vi "Source A.vi"() -> ()   [LabVIEW 2016, in "beamline sections.lvlib"]
doc: "This vi allows the user to control the beamline elements on the high voltage deck. It uses the GRoup3 controllers to access all three high voltage decks. The preacc and injector image faraday cup are controlled by the low end compact rio"
uses:
  beamline sections.lvlib
  Users/wymanm/Desktop/Control computer - Copy/control/control vi/ion Source/Ion Source/ion source llb.lvlib
panel:
  in  "Tab Control":enum32{"Controls", "Readbacks"}(tab)
  out "Boolean":bool
  in  "Oven i":dbl
  in  "Y Steerer":dbl(knob) scale=-500.0..300.0
  in  "Pre-Acc":dbl(knob) scale=60.0..63.0
  in  "source 2 Einzel":dbl(knob) scale=4.0..10.0
  in  "X Steerer":dbl(knob) scale=300.0..-300.0
  in  "Source 1 Einzel":dbl(knob) scale=8.0..12.0
  in  "Extractor p":dbl(knob) scale=20.0..26.0
  in  "Immersion Lens":dbl(knob) scale=0.0..1.0
  out "Einzel 2":bool
  out "Cathode":bool
  out "Extractor":bool
  out "Oven":bool
  out "Immersion lens":bool
  out "Einzel 1":bool
  out "Steerer":bool
  out "Pre acc":bool=TRUE
  in  "Cathode vol":dbl(knob) scale=0.0..10.0
  out "Cathode  cluster":T1 {"Cathode" format="%#_3g"; "Cathode\nVoltage" format="%#.2g"; "Cathode \nCurrent" format="%#.2g"}
  out "Extractor  cluster":T2 {"Extractor" format="%#_3g"; "Extractor \nVoltage" format="%#.2g"; "Extractor\n Current" format="%#.2g"}
  out "Immersion Lens  cluster":T3 {"Immersion Lens" format="%#_3g"; "Immersion Lens\nCurrent" format="%#.2g"; "Immersion Lens\nVoltage" format="%#.2g"}
  in  "stop":bool
  out "Oven cluster":T4 {"Oven V" format="%#.2g"; "Oven power" format="%#.2g"; "Oven  I readback" format="%#.2g"; "Oven Current\n Set point" format="%#.2g"}
  out "Einzel 1  cluster":T5 {"Einzel 1\nVoltage" format="%#.2g"; "Einzel \nCurrent" format="%#.2g"}
  out "Source Steerer cluster":T6 {"X steerer" format="%#.2g"; "Y Steerer" format="%#.2g"}
  out "Einzel 2  cluster":T7 {"Einzel 2\nvoltage" format="%#.2g"; "Einzel 2 \nCurrent" format="%#.2g"}
  out "Preacc cluster":T8 {"Pre-acc Voltage" format="%#.2g"; "Pre-acc current" format="%#.2g"}
  out "Cryo pump":T9
  out "Ion gauge Cluster 1":T10
  out "cathode on?":bool
  out "sample change finished change":bool
  out "holder position":bool
  out "cathode on":bool
  out "chop voltage":dbl
  in  "reset oven":bool
  out "Ion Source Readbacks":dbl[][](array[numeric])
  out "Ion Source":dbl[][](array[numeric])
  out "Oven":dbl[](array[numeric])
  out "Einzel":dbl[](array[numeric])
  out "pre-acc set":dbl format="%#_3g"
  out "Pre-acc Voltage":dbl format="%#_3g"
  out "Pre-acc current":dbl format="%#_3g"
  out "inj cup out":bool
  out "Output Current":dbl format="%.4f"
  out "Output Power":dbl format="%.4f"
  out "Output Voltage":dbl format="%.4f"
  out "error out 2":errorcluster
  out "Read Set Current":dbl format="%.4f"
  out "Read Set Voltage":dbl format="%.4f"
  out "error out":errorcluster
  out "ID responce":string
  out "Address \"OK\"":string
  in  "Einzel 1  cluster 2":T5 {"Einzel 1\nVoltage" format="%#.2g"; "Einzel \nCurrent" format="%#.2g"}
  # "red is in the beamline\nblue is out of the beamline"
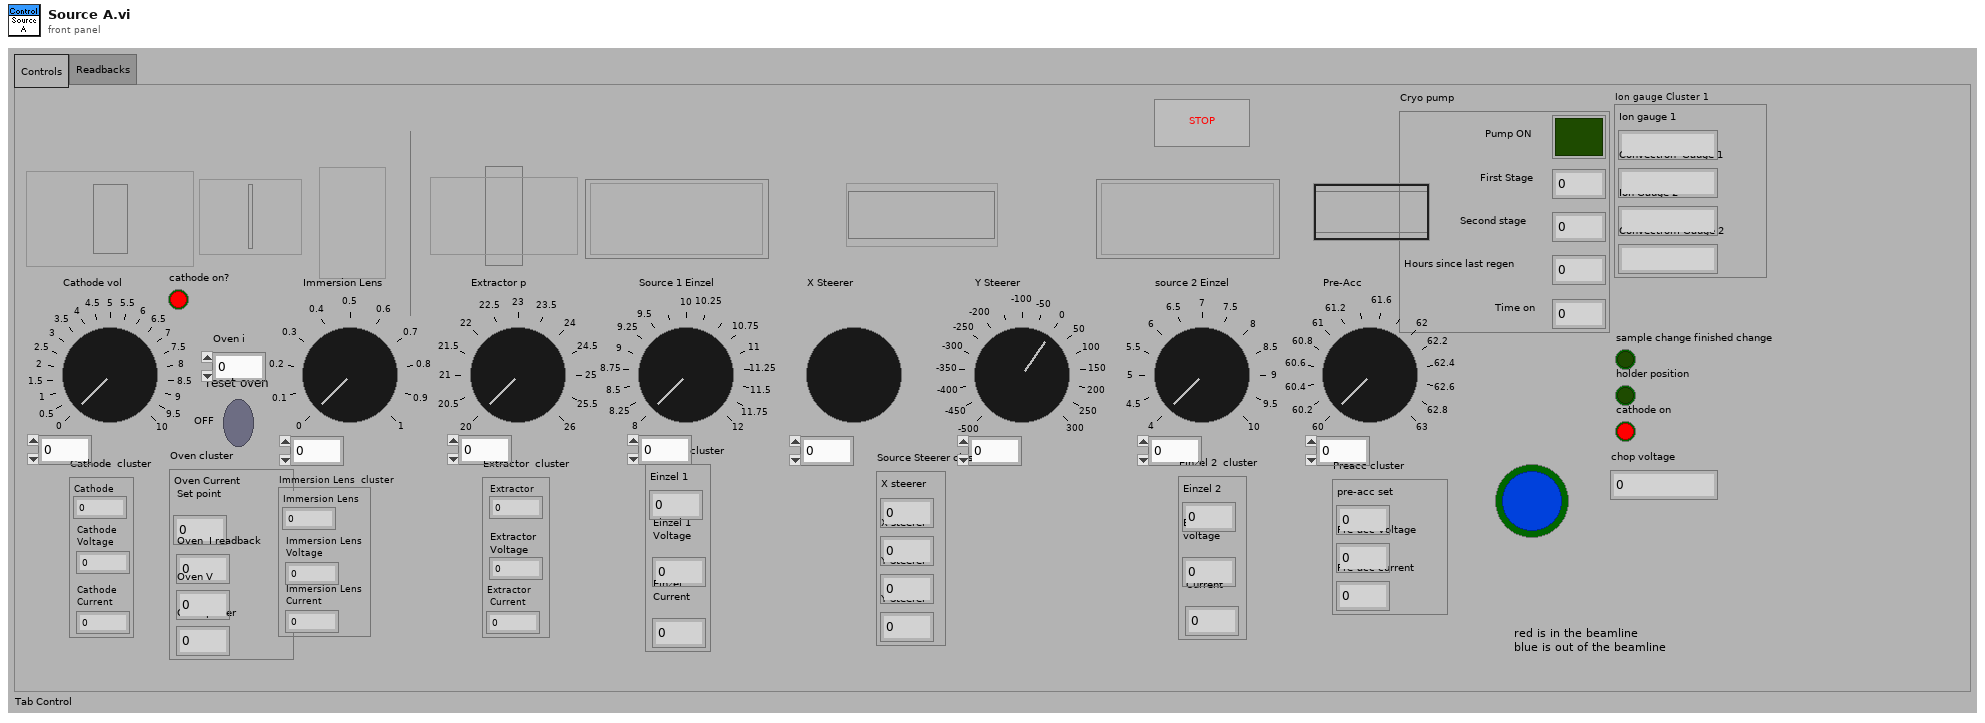
[diagram p1: front panel]
types:
  T1 = cluster{"Cathode":dbl, "Cathode\nVoltage":dbl, "Cathode \nCurrent":dbl}
  T2 = cluster{"Extractor":dbl, "Extractor \nVoltage":dbl, "Extractor\n Current":dbl}
  T3 = cluster{"Immersion Lens":dbl, "Immersion Lens\nCurrent":dbl, "Immersion Lens\nVoltage":dbl}
  T4 = cluster{"Oven  I readback":dbl, "Oven Current\n Set point":dbl, "Oven power":dbl, "Oven V ":dbl}
  T5 = cluster{"Einzel 1":dbl, "Einzel 1\nVoltage":dbl, "Einzel \nCurrent":dbl}
  T6 = cluster{"X steerer":dbl, "X steerer":dbl, "Y Steerer":dbl, "Y Steerer":dbl}
  T7 = cluster{"Einzel 2":dbl, "Einzel 2\nvoltage":dbl, "Einzel 2 \nCurrent":dbl}
  T8 = cluster{"pre-acc set":dbl, "Pre-acc Voltage":dbl, "Pre-acc current":dbl}
  T9 = cluster{"First Stage":dbl, "Second stage":dbl, "Hours since last regen":dbl, "Pump ON":bool, "Time on":dbl}
  T10 = cluster{"Ion gauge 1":string, "Convectron  Gauge 1 ":string, "Ion Gauge 2":string, "Convectrom Gauge 2":string}
  T11 = typedef "main.lvlib/saveload.ctl" = cluster{"OK Button":bool, "OK Button 2":bool, "OK Button 3":bool, "OK Button 4":bool}
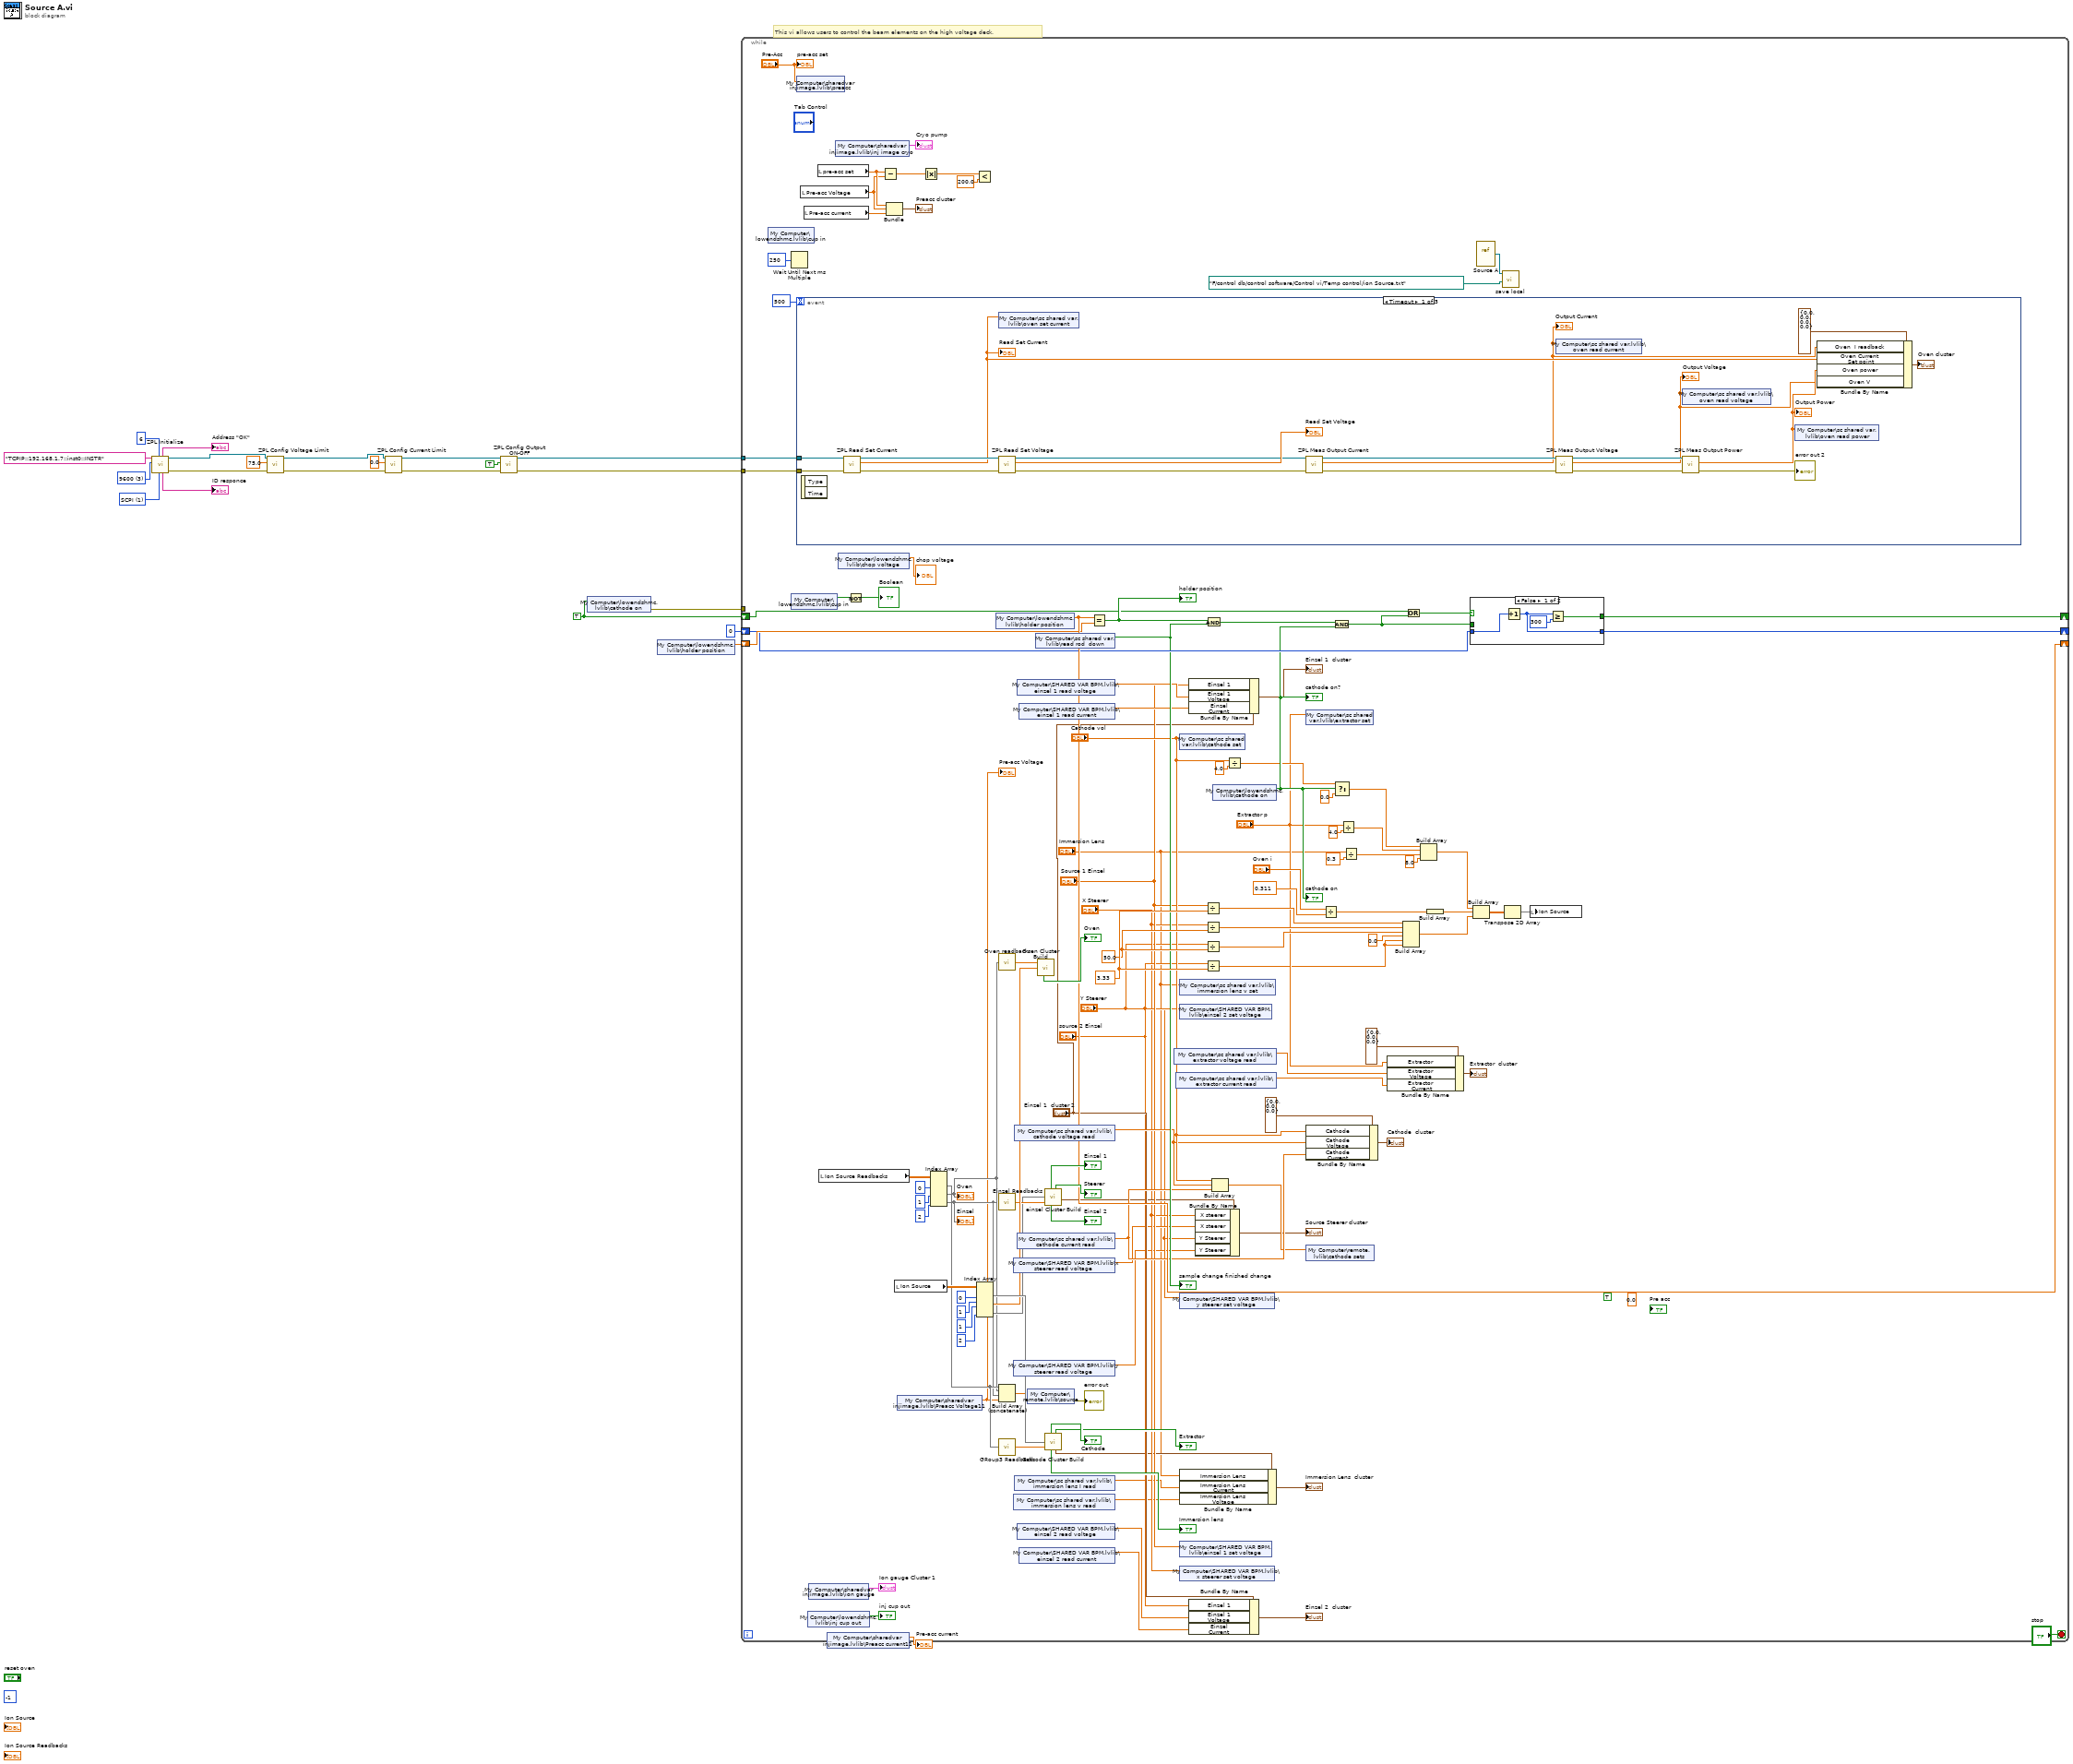
[diagram p0: block diagram]
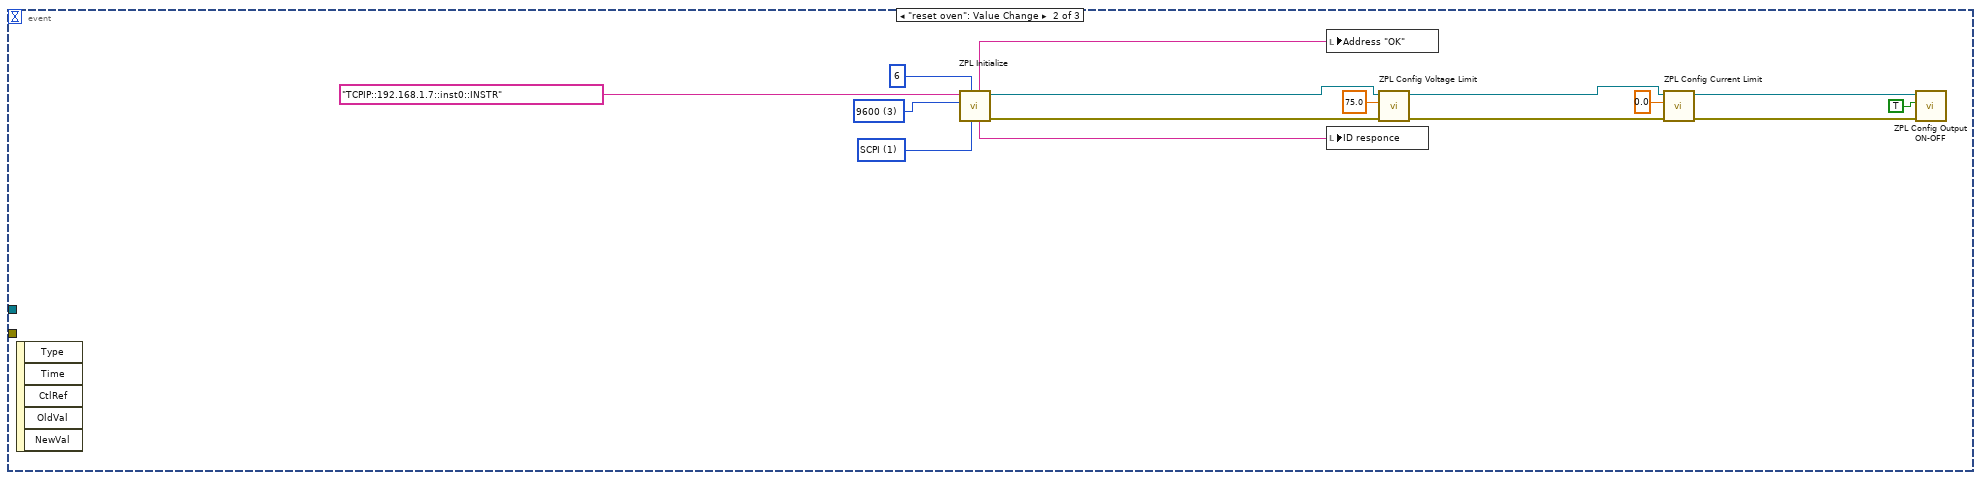
[diagram p2: hidden frame]
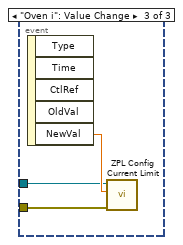
[diagram p3: hidden frame]
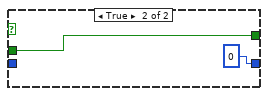
[diagram p4: hidden frame]
diagram:
  w17 = 3 items=["1200", "2400", "4800", "9600", "19200", "38400", "57600", "115200"] ("Baud Rate")
  w16 = i16 1 items=["GEN", "SCPI"] ("Language Selector")
  w18 = TRUE ("cathode on")
  (unwired) -1
  # "This vi allows users to control the beam elements on the high voltage deck."
  n1 = call "ZPL Initialize.vi"("Language Selector"=w16, "Address"=i16 6, "Baud Rate"=w17, "VISA"="TCPIP::192.168.1.7::inst0::INSTR" ("format string")) -> ("error out"=w7:errorcluster, "VISA  out"=w8:refnum<visa-resource-name>, "ID responce"=→"ID responce":string, "Address \"OK\""=→"Address \"OK\"":string)  [unwired: 4 in]
  n2 = call "ZPL Config Voltage Limit.vi"("error"=w7, "Voltage Limit"=75.0, "VISA"=w8) -> ("error out"=w9:errorcluster, "VISA out"=w10:refnum<visa-resource-name>)  [unwired: 7 in]
  n3 = call "ZPL Config Current Limit.vi"("error"=w9, "Current Limit"=0.0, "VISA"=w10) -> ("error out"=w13:errorcluster, "VISA out"=w12:refnum<visa-resource-name>)  [unwired: 7 in]
  n4 = call "ZPL Config Output ON-OFF.vi"("error"=w13, "Output ON"=TRUE, "VISA"=w12) -> ("error out"=w4:errorcluster, "VISA out"=w5:refnum<visa-resource-name>)  [unwired: 7 in]
  n5 = shared-variable "My Computer\\lowendshmc.lvlib\\cathode on"(w18) -> (error out=w21:errorcluster)  [unwired: 1 in]
  n6 = shared-variable "My Computer\\lowendshmc.lvlib\\holder position"() -> (w20:dbl)  [unwired: 1 in, 1 out]
  n7 = while {
    tunnel: w21 -> [_]
    shift-right: [w73] -> _
    shift-left: w20 -> [w72]
    shift-right: [w66] -> _
    shift-left: w18 -> [w60]
    shift-right: [w67] -> _
    shift-left: 0 ("index of element") -> [w68]
    tunnel: w5 -> [w43]
    tunnel: w4 -> [w42]
    stop <- "stop" stop-if-true
    (unwired) TRUE ("s")
    w101 = 50.0 ("y")
    w102 = 3.33 ("y")
    (unwired) 0.0 ("element")
    n8 = shared-variable "My Computer\\lowendshmc.lvlib\\cup in"() -> ()  [unwired: 1 in, 2 out]
    n9 = Wait Until Next ms Multiple(millisecond multiple=u32 250) -> ()  [unwired: 1 out]
    n10 = shared-variable "My Computer\\lowendshmc.lvlib\\cup in"() -> (w64:bool)  [unwired: 1 in, 1 out]
    n11 = shared-variable "My Computer\\sharedvar injimage.lvlib\\preacc"("Pre-Acc") -> ()  [unwired: 1 in, 1 out]
    n12 = event shown="[0] Timeout" {
      selector: _ -> [_ _ _]
      dyn-events: _ -> [_ _ _]
      timeout: 500 -> [_ _ _]
      tunnel: w43 -> [w147 _ w173]
      tunnel: w42 -> [w146 _ w174]
      event Timeout {
        n13 = event-data() -> ()  [unwired: 1 in, 2 out]
        n14 = call "ZPL Read Set Current.vi"("error"=w146, "VISA"=w147) -> ("error out"=w157:errorcluster, "Read Set Current"=w143:dbl, "VISA out"=w156:refnum<visa-resource-name>)  [unwired: 7 in]
        "Read Set Current" <- w143
        n15 = shared-variable "My Computer\\sc shared var.lvlib\\oven set current"(w143) -> ()  [unwired: 1 in, 1 out]
        n16 = call "ZPL Read Set Voltage.vi"("error"=w157, "VISA"=w156) -> ("error out"=w153:errorcluster, "Read Set Voltage"=→"Read Set Voltage":dbl, "VISA out"=w154:refnum<visa-resource-name>)  [unwired: 7 in]
        n17 = call "ZPL Meas Output Current.vi"("error"=w153, "VISA"=w154) -> ("error out"=w151:errorcluster, "Output Current"=w141:dbl, "VISA out"=w152:refnum<visa-resource-name>)  [unwired: 7 in]
        "Output Current" <- w141
        n18 = shared-variable "My Computer\\sc shared var.lvlib\\oven read current"(w141) -> ()  [unwired: 1 in, 1 out]
        n19 = call "ZPL Meas Output Voltage.vi"("error"=w151, "VISA"=w152) -> ("error out"=w149:errorcluster, "Output Voltage"=w140:dbl, "VISA out"=w150:refnum<visa-resource-name>)  [unwired: 7 in]
        "Output Voltage" <- w140
        n20 = shared-variable "My Computer\\sc shared var.lvlib\\oven read voltage"(w140) -> ()  [unwired: 1 in, 1 out]
        n21 = call "ZPL Meas Output Power.vi"("error"=w149, "VISA"=w150) -> ("error out"=→"error out 2":errorcluster, "Output Power"=w142:dbl)  [unwired: 7 in, 1 out]
        "Output Power" <- w142
        n22 = shared-variable "My Computer\\sc shared var.lvlib\\oven read power"(w142) -> ()  [unwired: 1 in, 1 out]
        n23 = Bundle By Name(cluster=T4 {"Oven  I readback"=0.0, "Oven Current\n Set point"=0.0, "Oven power"=0.0, "Oven V "=0.0} ("Oven cluster"), "Oven  I readback"=w141, "Oven Current\n Set point"=w143, "Oven power"=w142, "Oven V"=w140) -> (→"Oven cluster":T4)
      }
      event "reset oven": Value Change {
        w161 = 3 items=["1200", "2400", "4800", "9600", "19200", "38400", "57600", "115200"] ("Baud Rate")
        w162 = i16 1 items=["GEN", "SCPI"] ("Language Selector")
        n24 = event-data() -> ()  [unwired: 1 in, 5 out]
        n25 = call "ZPL Initialize.vi"("Language Selector"=w162, "Address"=i16 6, "Baud Rate"=w161, "VISA"="TCPIP::192.168.1.7::inst0::INSTR" ("format string")) -> ("error out"=w170:errorcluster, "VISA  out"=w169:refnum<visa-resource-name>, "ID responce"=w158:string, "Address \"OK\""=w159:string)  [unwired: 4 in]
        n26 = local write "Address \"OK\""(w159) -> ()
        n27 = local write "ID responce"(w158) -> ()
        n28 = call "ZPL Config Voltage Limit.vi"("error"=w170, "Voltage Limit"=75.0, "VISA"=w169) -> ("error out"=w168:errorcluster, "VISA out"=w167:refnum<visa-resource-name>)  [unwired: 7 in]
        n29 = call "ZPL Config Current Limit.vi"("error"=w168, "Current Limit"=0.0, "VISA"=w167) -> ("error out"=w164:errorcluster, "VISA out"=w165:refnum<visa-resource-name>)  [unwired: 7 in]
        n30 = call "ZPL Config Output ON-OFF.vi"("error"=w164, "Output ON"=TRUE, "VISA"=w165) -> ()  [unwired: 7 in, 2 out]
      }
      event "Oven i": Value Change {
        n31 = event-data() -> ("NewVal"=w175:dbl)  [unwired: 1 in, 4 out]
        n32 = call "ZPL Config Current Limit.vi"("error"=w174, "Current Limit"=w175, "VISA"=w173) -> ()  [unwired: 7 in, 2 out]
      }
    }
    n33 = local read "Pre-acc Voltage"() -> (w112:dbl)
    n34 = local read "Pre-acc current"() -> (w115:dbl)
    n35 = shared-variable "My Computer\\lowendshmc.lvlib\\inj cup out"() -> (→"inj cup out":bool)  [unwired: 1 in, 1 out]
    n36 = shared-variable "My Computer\\sharedvar injimage.lvlib\\ion gauge"() -> (→"Ion gauge Cluster 1":cluster{string, string, string, string})  [unwired: 1 in, 1 out]
    n37 = local read "pre-acc set"() -> (w113:dbl)
    n38 = local read "Ion Source Readbacks"() -> (w134:dbl[][])
    n39 = shared-variable "My Computer\\sharedvar injimage.lvlib\\Preacc current11"() -> (→"Pre-acc current":dbl)  [unwired: 1 in, 1 out]
    n40 = shared-variable "My Computer\\sharedvar injimage.lvlib\\inj image cryo"() -> (→"Cryo pump":T9)  [unwired: 1 in, 1 out]
    n41 = shared-variable "My Computer\\lowendshmc.lvlib\\chop voltage"() -> (→"chop voltage":dbl)  [unwired: 1 in, 1 out]
    n42 = Not(x=w64) -> (.not. x?=→"Boolean":bool)
    n43 = Subtract(x=w113, y=w112) -> (x-y=w110:dbl)
    n44 = Bundle("pre-acc set"=w113, "Pre-acc Voltage"=w112, "Pre-acc current"=w115) -> (→"Preacc cluster":T8)  [unwired: 1 out]
    n45 = local read "Ion Source"() -> (w132:dbl[][])
    n46 = shared-variable "My Computer\\sharedvar injimage.lvlib\\Preacc Voltage11"() -> (w76:dbl)  [unwired: 1 in, 1 out]
    "Pre-acc Voltage" <- w76
    n47 = Absolute Value(x=w110) -> (abs(x)=w109:dbl)
    n48 = Index Array(array=w134, index (col) #1=0 ("disabled index (col)"), index (col) #2=1 ("index (col)"), index (col) #3=2 ("index (col)")) -> (element #1=w79:dbl[], element #2=w78:dbl[], element #3=w77:dbl[])  [unwired: 3 in]
    "Oven" <- w78
    "Einzel" <- w77
    n49 = Less?(x=w109, y=200.0) -> ()  [unwired: 1 out]
    n50 = Index Array(array=w132, index (col) #1=0 ("disabled index (col)"), index (row) #2=1 ("disabled index (row)"), index (col) #2=1 ("index (col)"), index (col) #3=2 ("index (col)")) -> (element #1=w128:dbl[], element #2=w122:dbl, element #3=w119:dbl[])  [unwired: 2 in]
    n51 = shared-variable "My Computer\\lowendshmc.lvlib\\holder position"() -> (w73:dbl)  [unwired: 1 in, 1 out]
    n52 = call "Oven readbacks.vi"("Oven  Rack Readbacks"=w78) -> ("Oven Current readback"=w123:dbl)
    n53 = call "Einzel Readbacks.vi"("Einzel  Rack Readbacks"=w77) -> ("Scaled Einzel Readbacks"=w120:dbl[])
    n54 = Build Array (concatenate)(w79, w78, w77, w76) -> (w75:dbl[])
    n55 = call "GRoup3 Readbacks.vi"("Cathode Rack Readbacks"=w79) -> ("Cathode Rack Readbacks"=w133:dbl[])
    n56 = shared-variable "My Computer\\SHARED VAR BPM.lvlib\\x steerer read voltage"() -> (w29:dbl)  [unwired: 1 in, 1 out]
    n57 = shared-variable "My Computer\\SHARED VAR BPM.lvlib\\y steerer read voltage"() -> (w27:dbl)  [unwired: 1 in, 1 out]
    n58 = shared-variable "My Computer\\sc shared var.lvlib\\immersion lens v read"() -> (w22:dbl)  [unwired: 1 in, 1 out]
    n59 = shared-variable "My Computer\\sc shared var.lvlib\\cathode voltage read"() -> (w48:dbl)  [unwired: 1 in, 1 out]
    n60 = shared-variable "My Computer\\sc shared var.lvlib\\immersion lens I read"() -> (w23:dbl)  [unwired: 1 in, 1 out]
    n61 = shared-variable "My Computer\\SHARED VAR BPM.lvlib\\einzel 1 read voltage"() -> (w41:dbl)  [unwired: 1 in, 1 out]
    n62 = shared-variable "My Computer\\sc shared var.lvlib\\cathode current read"() -> (w47:dbl)  [unwired: 1 in, 1 out]
    n63 = shared-variable "My Computer\\SHARED VAR BPM.lvlib\\einzel 2 read voltage"() -> (w34:dbl)  [unwired: 1 in, 1 out]
    n64 = shared-variable "My Computer\\SHARED VAR BPM.lvlib\\einzel 1 read current"() -> (w40:dbl)  [unwired: 1 in, 1 out]
    n65 = shared-variable "My Computer\\SHARED VAR BPM.lvlib\\einzel 2 read current"() -> (w33:dbl)  [unwired: 1 in, 1 out]
    n66 = shared-variable "My Computer\\remote.lvlib\\source"(w75) -> (error out=→"error out":errorcluster)  [unwired: 1 in]
    n67 = shared-variable "My Computer\\sc shared var.lvlib\\read rod  down"() -> (w59:bool)  [unwired: 1 in, 1 out]
    "sample change finished change" <- w59
    n68 = call "Oven Cluster Build.vi"("Oven readback"=w123, "Oven Current Set point"=w122) -> ("Oven  range"=→"Oven":bool)  [unwired: 8 out]
    n69 = call "einzel Cluster Build.vi"("Einzel rack"=w119, "Einzel Rack Readbacks"=w120) -> ("Einzel 1 range"=→"Einzel 1":bool, "Einzel 2  range"=→"Einzel 2":bool, "Source steerer range"=→"Steerer":bool, "Source Steerer cluster"=w32:T6)  [unwired: 5 out]
    n70 = call "Cathode Cluster Build.vi"("Ion Source"=w128, "Cathode Rack Readbacks"=w133) -> ("Cathode range"=→"Cathode":bool, "Immersion lens  range"=→"Immersion lens":bool, "Extractor range"=→"Extractor":bool, "Immersion Lens  cluster"=w26:T3)  [unwired: 5 out]
    n71 = Equal?(x=w73, y=w72) -> (x = y?=w71:bool)
    "holder position" <- w71
    n72 = shared-variable "My Computer\\sc shared var.lvlib\\extractor voltage read"() -> (w53:dbl)  [unwired: 1 in, 1 out]
    n73 = shared-variable "My Computer\\sc shared var.lvlib\\extractor current read"() -> (w51:dbl)  [unwired: 1 in, 1 out]
    n74 = shared-variable "My Computer\\sc shared var.lvlib\\cathode set"("Cathode vol") -> ()  [unwired: 1 in, 1 out]
    n75 = shared-variable "My Computer\\sc shared var.lvlib\\immersion lens v set"("Immersion Lens") -> ()  [unwired: 1 in, 1 out]
    n76 = shared-variable "My Computer\\SHARED VAR BPM.lvlib\\einzel 2 set voltage"("source 2 Einzel") -> ()  [unwired: 1 in, 1 out]
    n77 = shared-variable "My Computer\\SHARED VAR BPM.lvlib\\y steerer set voltage"("Y Steerer") -> ()  [unwired: 1 in, 1 out]
    n78 = Bundle By Name(cluster=w26, "Immersion Lens"="Immersion Lens", "Immersion Lens\nCurrent"=w23, "Immersion Lens\nVoltage"=w22) -> (→"Immersion Lens  cluster":T3)
    n79 = shared-variable "My Computer\\SHARED VAR BPM.lvlib\\einzel 1 set voltage"("Source 1 Einzel") -> ()  [unwired: 1 in, 1 out]
    n80 = shared-variable "My Computer\\SHARED VAR BPM.lvlib\\x steerer set voltage"("X Steerer") -> ()  [unwired: 1 in, 1 out]
    n81 = Bundle By Name(cluster="Einzel 1  cluster 2", "Einzel 1"="Source 1 Einzel", "Einzel 1\nVoltage"=w41, "Einzel \nCurrent"=w40) -> (→"Einzel 1  cluster":T5)
    n82 = Bundle By Name(cluster="Einzel 1  cluster 2", "Einzel 1"="source 2 Einzel", "Einzel 1\nVoltage"=w34, "Einzel \nCurrent"=w33) -> (→"Einzel 2  cluster":T5)
    n83 = Bundle By Name(cluster=w32, "X steerer"="X Steerer", "X steerer"=w29, "Y Steerer"="Y Steerer", "Y Steerer"=w27) -> (→"Source Steerer cluster":T6)
    n84 = Divide(x="Source 1 Einzel", y=w102) -> (x/y=w98:dbl)
    n85 = Divide(x="X Steerer", y=w101) -> (x/y=w97:dbl)
    n86 = Divide(x="Y Steerer", y=w101) -> (x/y=w96:dbl)
    n87 = Divide(x="source 2 Einzel", y=w102) -> (x/y=w45:dbl)
    n88 = And(x=w71, y=w59) -> (x .and. y?=w70:bool)
    n89 = Build Array("Cathode vol", w48, w47) -> (w46:dbl[])
    n90 = shared-variable "My Computer\\lowendshmc.lvlib\\cathode on"() -> (w58:bool)  [unwired: 1 in, 1 out]
    "cathode on?" <- w58
    "cathode on" <- w58
    n91 = Divide(x="Cathode vol", y=4.0) -> (x/y=w57:dbl)
    n92 = shared-variable "My Computer\\sc shared var.lvlib\\extractor set"("Extractor p") -> ()  [unwired: 1 in, 1 out]
    n93 = Bundle By Name(cluster=T1 {"Cathode"=0.0, "Cathode\nVoltage"=0.0, "Cathode \nCurrent"=0.0} ("Cathode  cluster"), "Cathode"="Cathode vol", "Cathode\nVoltage"=w48, "Cathode \nCurrent"=w47) -> (→"Cathode  cluster":T1)
    n94 = shared-variable "My Computer\\remote.lvlib\\cathode sets"(w46) -> ()  [unwired: 1 in, 1 out]
    n95 = Divide(x="Oven i", y=0.311) -> (x/y=w95:dbl)
    n96 = And(x=w70, y=w58) -> (x .and. y?=w65:bool)
    n97 = Select(t=w57, s=w58, f=0.0) -> (s? t:f=w61:dbl)
    n98 = Divide(x="Extractor p", y=4.0) -> (x/y=w90:dbl)
    n99 = Divide(x="Immersion Lens", y=0.3) -> (x/y=w91:dbl)
    n100 = Bundle By Name(cluster=T2 {"Extractor"=0.0, "Extractor \nVoltage"=0.0, "Extractor\n Current"=0.0} ("Extractor  cluster"), "Extractor"="Extractor p", "Extractor \nVoltage"=w53, "Extractor\n Current"=w51) -> (→"Extractor  cluster":T2)
    n101 = Build Array(w98, w97, w96, 0.0 ("element"), w45, w45) -> (w80:dbl[])
    n102 = Or(x=w60, y=w65) -> (x .or. y?=w69:bool)
    n103 = Build Array(w61, w90, w91, 8.0 ("element")) -> (w82:dbl[])
    n104 = Build Array(w95) -> (w81:dbl[])
    n105 = case shown="False" w69 {
      tunnel: w68 -> [w179 _]
      tunnel: [w178 0] -> w67
      tunnel: [w176 w180] -> w66
      tunnel: w65 -> [_ w180]
      frame False {
        n106 = Increment(x=w179) -> (x+1=w178:i32)
        n107 = Greater Or Equal?(x=w178, y=300) -> (x >= y?=w176:bool)
      }
      frame True {
      }
    }
    n108 = Build Array(w82, w81, w80) -> (w94:dbl[][])
    n109 = vi-ref "Source A.vi"() -> (w108:refnum<vi>)
    n110 = call "save local.vi"("file path (use dialog)"=path "F:/control db/control software/Control vi/Temp control/ion Source.txt", "VI Refnum"=w108) -> ("Ring"=w107:T11)  [unwired: 1 in, 1 out]
    n111 = Transpose 2D Array(2D array=w94) -> (transposed array=w93:dbl[][])
    n112 = local write "Ion Source"(w93) -> ()
    "pre-acc set" <- "Pre-Acc"
  }
